vi "Delete Previous Report.vi"(8 "error in (no error)":errorcluster, 9 "ImageFolder":string="Images", 10 "ReportName":string="Lumberjack_Report.html", 11 "outputFolder in":path=path "C:/Users/dallis/OneDrive - Velico Medical/Documents/Personal/LabVIEW Coding Projects/Lumberjack/docs/HTMLReport") -> (0 "error out":errorcluster, 1 "imagesFolder":path=path "C:/Users/dallis/OneDrive - Velico Medical/Documents/Personal/LabVIEW Coding Projects/Lumberjack/docs/HTMLReport", 2 "reportFile":path=path "C:/Users/dallis/OneDrive - Velico Medical/Documents/Personal/LabVIEW Coding Projects/Lumberjack/docs/HTMLReport", 3 "outputFolder out":path=path "C:/Users/dallis/OneDrive - Velico Medical/Documents/Personal/LabVIEW Coding Projects/Lumberjack/docs/HTMLReport")   [LabVIEW 2026]
doc: "Update with test documentation"
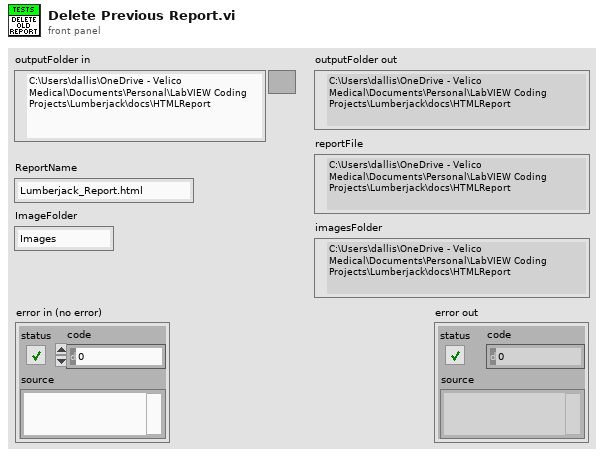
[diagram p1: front panel]
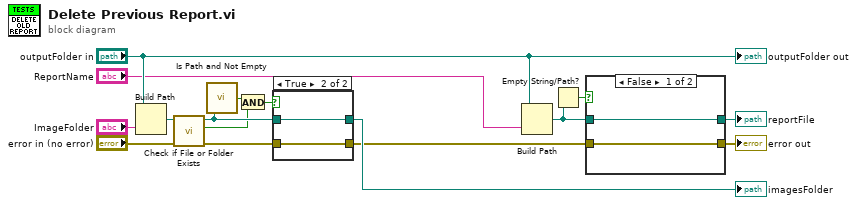
[diagram p0: block diagram]
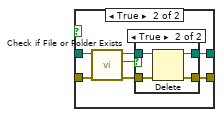
[diagram p2: hidden frame]
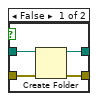
[diagram p4: hidden frame]
diagram:
  n1 = Build Path(base path="outputFolder in", name or relative path="ImageFolder") -> (appended path=w16:path)
  n2 = call <vilib>:"Check if File or Folder Exists.vi"("error in (no error)"="error in (no error)", "path"=w16) -> ("error out"=w14:errorcluster, "file or folder exists?"=w12:bool, "dup path"=w15:path)  [unwired: 7 in]
  n3 = call <vilib>:"Is Path and Not Empty.vi"("path"=w15) -> ("Is Path and Not Empty?"=w13:bool)  [unwired: 4 in]
  n4 = And(x=w13, y=w12) -> (x .and. y?=w11:bool)
  n5 = case shown="True" w11 {
    tunnel: w15 -> [w20 w22]
    tunnel: w14 -> [w19 w21]
    tunnel: [w18 w21] -> w6
    tunnel: [w17 w22] -> w8
    frame False {
      n6 = Create Folder(path (use dialog)=w20, error in=w19) -> (created path=w17:path, error out=w18:errorcluster)  [unwired: 1 in, 1 out]
    }
    frame True {
    }
  }
  "imagesFolder" <- w8
  n7 = Build Path(base path="outputFolder in", name or relative path="ReportName") -> (appended path=w10:path)
  n8 = Empty String/Path?(string/path=w10) -> (empty?=w9:bool)
  n9 = case shown="False" w9 {
    tunnel: w10 -> [w24 w30]
    tunnel: [w23 w31] -> w4
    tunnel: [w24 w26] -> w5
    tunnel: w6 -> [w23 w25]
    frame False {
    }
    frame True {
      n10 = call <vilib>:"Check if File or Folder Exists.vi"("error in (no error)"=w25, "path"=w30) -> ("error out"=w29:errorcluster, "file or folder exists?"=w27:bool, "dup path"=w28:path)  [unwired: 7 in]
      n11 = case shown="True" w27 {
        tunnel: [w33 w37] -> w31
        tunnel: w29 -> [w33 w36]
        tunnel: w28 -> [w32 w35]
        tunnel: [w32 w34] -> w26
        frame False {
        }
        frame True {
          n12 = Delete(path (use dialog)=w35, error in=w36) -> (deleted path=w34:path, error out=w37:errorcluster)  [unwired: 3 in, 1 out]
        }
      }
    }
  }
  "error out" <- w4
  "reportFile" <- w5
  "outputFolder out" <- "outputFolder in"
